vi "Acquisition-Enter.vi"(0 "Logging queue element in":T2 {"Ref Dwell time (us)" format="%#.6g"; "Frame Size" items=["100X100"=100, "128X128"=128, "200X200"=200, "256X256"=256, "512X512"=512, "1024x1024"=1024, "2048x2048"=2048]; "Dwell time (us)" format="%#.6g"}, 5 "Imaging Protocol":T1, 7 "FPGA Ref":T5, 9 "Target number of points":u64, 11 "error in (no error)":errorcluster) -> (4 "Logging queue element out":T2 {"Ref Dwell time (us)" format="%#.6g"; "Frame Size" items=["100X100"=100, "128X128"=128, "200X200"=200, "256X256"=256, "512X512"=512, "1024x1024"=1024, "2048x2048"=2048]; "Dwell time (us)" format="%#.6g"}, 6 "Read at least # points":u32, 10 "Read at least # Ref points":u32, 15 "error out":errorcluster)   [LabVIEW 2017]
uses:
  RIG-SPECIFIC FILES/FPGA Refs/FPGA Ref.ctl
  Typedefs/Logging queue element.ctl
  Typedefs/Imaging Protocols enum.ctl
  Typedefs/Frame Size.ctl
  Typedefs/Acquired points count.ctl
  Typedefs/Read Write Enum.ctl
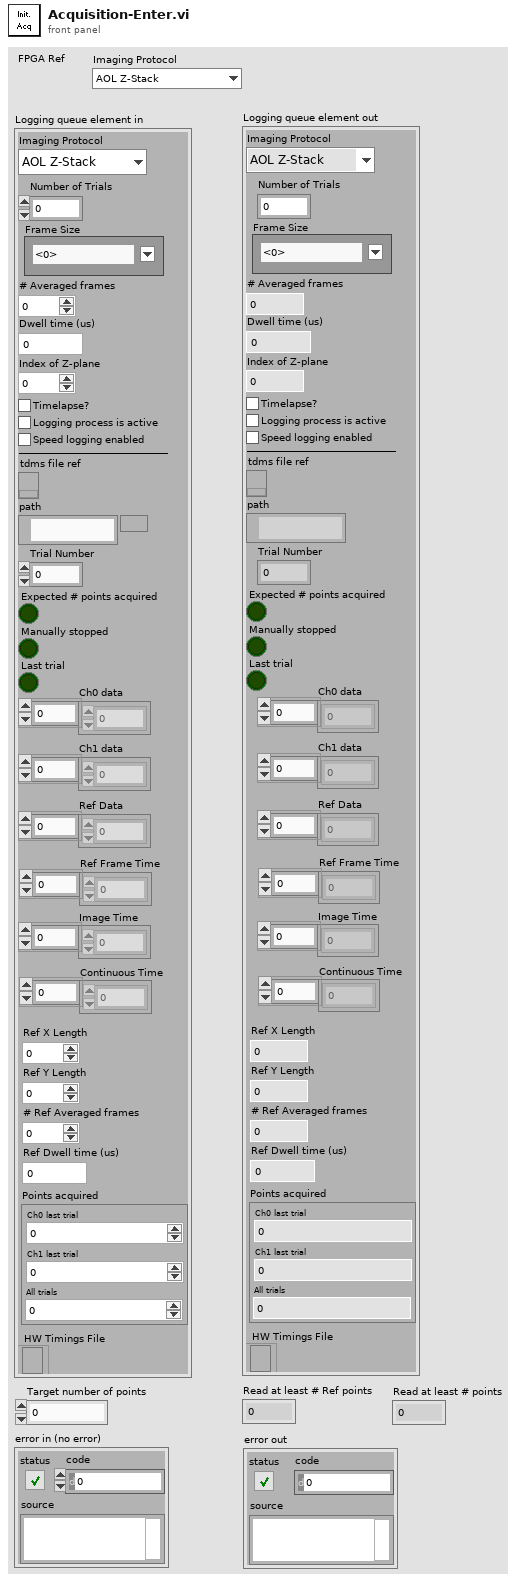
[diagram p1: front panel]
types:
  T1 = typedef "Imaging Protocols enum.ctl" = enum16{"AOL Z-Stack", "Motor Z Stack", "Functional Acquisition", "Single Plane Acquisition", "Volume Acquisition", "Live Imaging", "Live Plane Imaging", "Live Volume Imaging"}
  T2 = typedef "Logging queue element.ctl" = cluster{"Imaging Protocol":T1, "Number of Trials":u16, "Frame Size":T3, "# Averaged frames":u16, "Dwell time (us)":dbl, "Index of Z-plane":i32, "Timelapse?":bool, "Logging process is active":bool, "Speed logging enabled":bool, "tdms file ref":refnum<k34>, "path":path, "Trial Number":i32, "Expected # points acquired":bool, "Manually stopped":bool, "Last trial":bool, "Ch0 data":u32[], "Ch1 data":u32[], "Ref Data":u32[], "Ref Frame Time":u64[], "Image Time":u64[], "Continuous Time":u64[], "Ref X Length":u16, "Ref Y Length":u16, "# Ref Averaged frames":u16, "Ref Dwell time (us)":dbl, "Points acquired":T4, "HW Timings File":refnum<file>}
  T3 = typedef "Frame Size.ctl" = u16
  T4 = typedef "Acquired points count.ctl" = cluster{"Ch0 last trial":u64, "Ch1 last trial":u64, "All trials":u64}
  T5 = typedef "FPGA Ref.ctl" = refnum<k20>
  T6 = typedef "Read Write Enum.ctl" = enum16{"Read", "Write"}
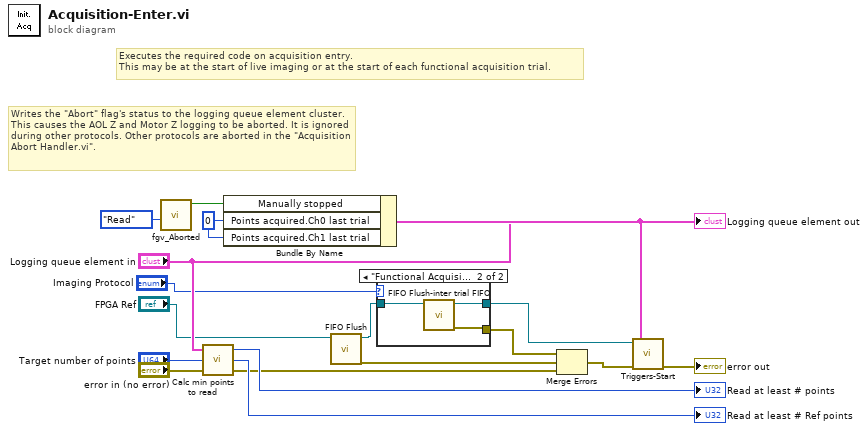
[diagram p0: block diagram]
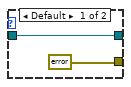
[diagram p2: hidden frame]
diagram:
  w18 = u32 0 ("Points acquired.Ch0 last trial")
  # "Writes the \"Abort\" flag's status to the logging queue element cluster. This causes the AOL Z and Motor Z logging to be aborted. It is ignored during other protocols. Other protocols are aborted in the \"Acquisition Abort Handler.vi\"."
  # "Executes the required code on acquisition entry.\nThis may be at the start of live imaging or at the start of each functional acquisition trial."
  n1 = call "fgv_Aborted.vi"("Function"=Read_Write_Enum."Read") -> ("Funct Acq Aborted?"=w9:bool)  [unwired: 9 in, 1 out]
  n2 = call "Calc min points to read.vi"("error in"="error in (no error)", "Target number of points"="Target number of points", "Logging queue element"="Logging queue element in") -> ("error out"=w1:errorcluster, "Read at least # Ref points"=→"Read at least # Ref points":u32, "Read at least # points"=→"Read at least # points":u32)
  n3 = Bundle By Name(cluster="Logging queue element in", "Manually stopped"=w9, "Points acquired.Ch0 last trial"=w18, "Points acquired.Ch1 last trial"=w18) -> (w17:T2)
  "Logging queue element out" <- w17
  n4 = call "FIFO Flush.vi"("FPGA VI Ref"="FPGA Ref") -> ("Error Out"=w8:errorcluster, "FPGA VI Reference Out"=w3:T5)  [unwired: 8 in, 1 out]
  n5 = case shown="\"Functional Acquisition\"" "Imaging Protocol" {
    tunnel: w3 -> [w20 w23]
    tunnel: [errorcluster {"status"=FALSE, "code"=0, "source"=""} ("error out") w22] -> w5
    tunnel: [w20 w21] -> w2
    frame Default {
    }
    frame "Functional Acquisition" {
      n6 = call "FIFO Flush-inter trial FIFO.vi"("FPGA VI Ref"=w23) -> ("error out"=w22:errorcluster, "FPGA VI Reference Out"=w21:T5)  [unwired: 9 in]
    }
  }
  n7 = Merge Errors(w5, w8, w1) -> (w7:errorcluster)
  n8 = call "Triggers-Start.vi"("Setup/Logging queue element"=w17, "error in (no error)"=w7, "FPGA Ref"=w2) -> ("error out"=→"error out":errorcluster)  [unwired: 8 in]
